vi "stage_waitforpiezo.vi"(8 "error in (no error)":errorcluster, 10 "Position":sgl, 11 "reference":refnum<k7>) -> (0 "error out":errorcluster, 3 "reference out":refnum<k7>)   [LabVIEW 2018]
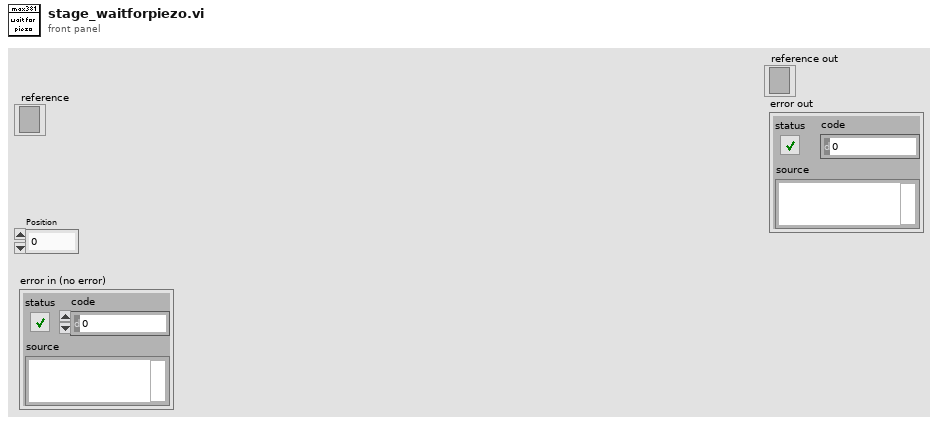
[diagram p1: front panel]
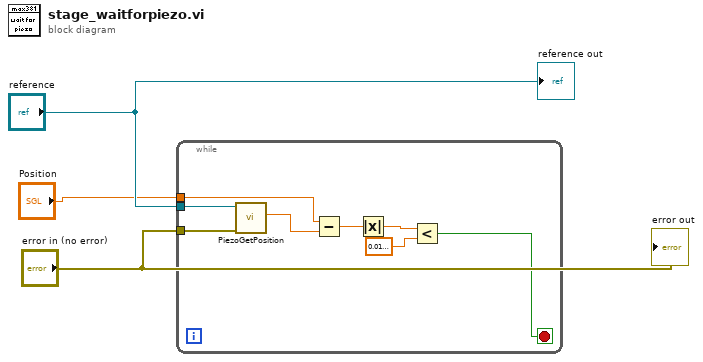
[diagram p0: block diagram]
diagram:
  n1 = while {
    tunnel: "reference" -> [w11]
    tunnel: "error in (no error)" -> [w10]
    tunnel: "Position" -> [w9]
    stop <- w4 stop-if-true
    n2 = call <userlib>:"PiezoGetPosition.vi"("error in (no error)"=w10, "reference"=w11) -> ("Position"=w8:sgl)  [unwired: 3 in, 2 out]
    n3 = Subtract(x=w9, y=w8) -> (x-y=w7:sgl)
    n4 = Absolute Value(x=w7) -> (abs(x)=w6:sgl)
    n5 = Less?(x=w6, y=sgl 0.02) -> (x < y?=w4:bool)
  }
  "reference out" <- "reference"
  "error out" <- "error in (no error)"
